vi "SPOL_temps_PB2.vi"() -> ()   [LabVIEW 2009]
uses:
  <vilib>/Utility/file.llb/Read From Spreadsheet File (string).vi
panel:
  in  "stop":bool
  in  "Select":bool
  in  "Plot":bool
  out "Housekeeping File":path caption="selected path"
  out "SPOL ATE Temperatures":T1(graph)={"[0]"=20.803, "[1]"=25.497, "[2]"=25.082, "[3]"=23.863, "[4]"=24.196, "[5]"=22.894, "[6]"=19.558, "[7]"=4.76, "[8]"=31.795, "[9]"=23.945, "[10]"=27.642, "[11]"=22.229, "[12]"=-999.0, "[13]"=21.308, "[14]"=25.608}
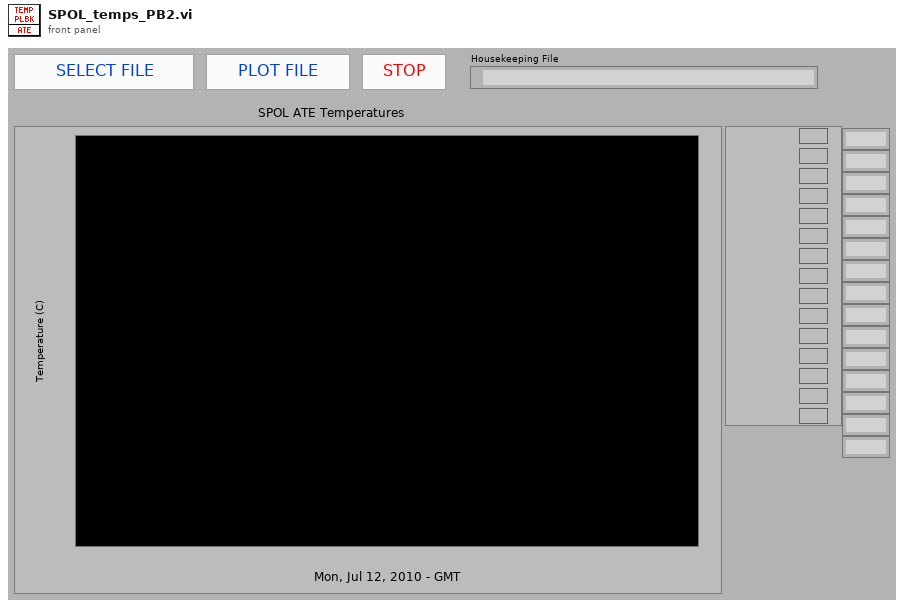
[diagram p1: front panel]
types:
  T1 = cluster{"[0]":dbl, "[1]":dbl, "[2]":dbl, "[3]":dbl, "[4]":dbl, "[5]":dbl, "[6]":dbl, "[7]":dbl, "[8]":dbl, "[9]":dbl, "[10]":dbl, "[11]":dbl, "[12]":dbl, "[13]":dbl, "[14]":dbl}
  T2 = cluster{"[0]":dbl, "[1]":dbl, "[2]":dbl, "[3]":dbl, "[4]":dbl, "[5]":dbl, "[6]":dbl, "[7]":dbl, "[8]":dbl, "[9]":dbl, "[10]":dbl, "[11]":dbl, "[12]":dbl, "[13]":dbl, "[14]":dbl}[]
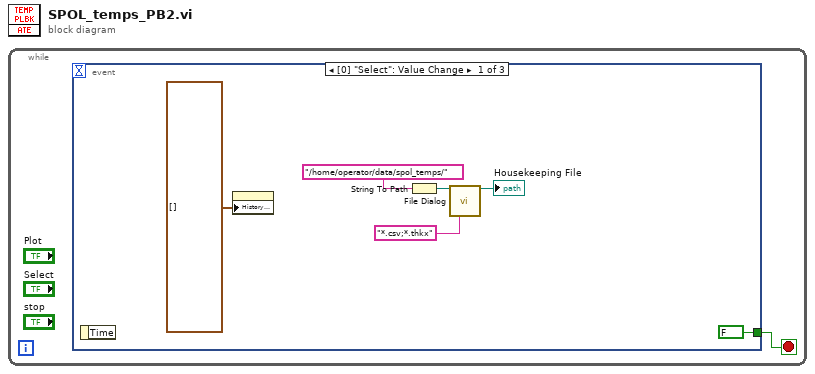
[diagram p0: block diagram]
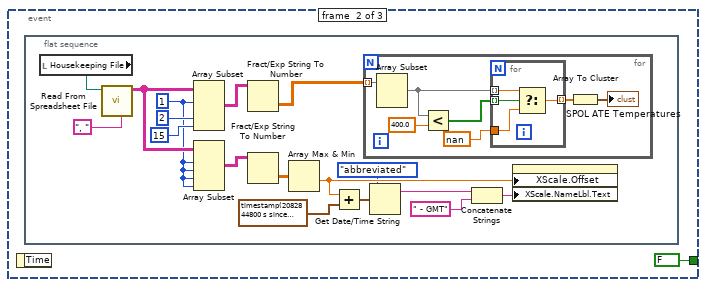
[diagram p2: hidden frame]
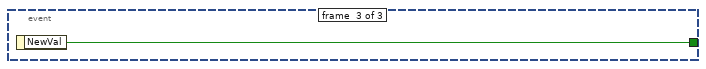
[diagram p3: hidden frame]
diagram:
  n1 = while {
    stop <- w1 stop-if-true
    n2 = event shown="[0] \"Select\": Value Change" {
      selector: _ -> [_ _ _]
      dyn-events: _ -> [_ _ _]
      timeout: _ -> [_ _ _]
      tunnel: [FALSE ("NewVal") FALSE w37] -> w1
      event #0 {
        n3 = event-data() -> ()  [unwired: 1 in, 1 out]
        n4 = property on="SPOL ATE Temperatures" class="WFChart (strict)"("History Data"=T2 []) -> ()  [unwired: 2 in, 2 out]
        n5 = String To Path(string="/home/operator/data/spol_temps/") -> (path=w5:path)
        n6 = call "File Dialog"("start path"=w5, "pattern (all files)"="*.csv;*.thkx") -> ("selected path"=→"Housekeeping File":path)  [unwired: 10 in, 3 out]
      }
      event #1 {
        n7 = event-data() -> ()  [unwired: 1 in, 1 out]
        n8 = flat-sequence {
          frame #0 {
            w17 = 1 ("index")
            n9 = local read "Housekeeping File"() -> (w25:path)
            n10 = call-poly <vilib>:"Read From Spreadsheet File.vi"("delimiter (\\t)"=", " ("delimiter (\\t)"), "file path (dialog if empty)"=w25) -> ("all rows"=w21:string[][])  [unwired: 5 in, 4 out]
            n11 = Array Subset(array=w21, index (row)=w17, index (col)=2 ("index"), length (col)=15 ("length")) -> (w24:string[][])  [unwired: 1 in]
            n12 = Array Subset(array=w21, index (row)=w17, length (row)=w17, index (col)=w17, length (col)=w17) -> (w20:string[][])
            n13 = Fract/Exp String To Number(string=w24) -> (number=w22:dbl[][])  [unwired: 3 in, 1 out]
            n14 = Fract/Exp String To Number(string=w20) -> (number=w16:dbl[][])  [unwired: 3 in, 1 out]
            n15 = Array Max & Min(array=w16) -> (min value=w15:dbl)  [unwired: 3 out]
            n16 = Add(x=w15, y=timestamp(2082844800 s since 1904-01-01)) -> (x+y=w13:timestamp)
            n17 = for {
              tunnel: w22 -> [w32] mode=indexing
              n18 = Array Subset(array=w32) -> (w28:dbl[])  [unwired: 2 in]
              n19 = Less?(x=w28, y=400.0 ("element")) -> (x < y?=w27:bool[])
              n20 = for {
                tunnel: w27 -> [w36] mode=indexing
                tunnel: w28 -> [w34] mode=indexing
                tunnel: nan ("number/path/refnum") -> [w35]
                tunnel: [w33] -> w29 mode=indexing
                n21 = Select(t=w34, s=w36, f=w35) -> (s? t:f=w33:dbl)
              }
              n22 = Array To Cluster(array=w29) -> (cluster=→"SPOL ATE Temperatures":T1)
            }
            n23 = Get Date/Time String(date format (0)=enum16{"short", "long", "abbreviated"}."abbreviated", seconds (now)=w13) -> (date string=w12:string)  [unwired: 1 in, 1 out]
            n24 = Concatenate Strings(w12, " - GMT" ("string")) -> (w11:string)
            n25 = property on="SPOL ATE Temperatures" class="WFChart (strict)"("XScale.Offset"=w15, "XScale.NameLbl.Text"=w11) -> ()  [unwired: 2 in, 2 out]
          }
        }
      }
      event #2 {
        n26 = event-data() -> ("NewVal"=w37:bool)  [unwired: 1 in]
      }
    }
  }
